vi "AlazarBusy.vi"(0 "Handle":u64, 1 "error in (no error)":errorcluster) -> (2 "Handle":u64, 3 "Busy":bool, 4 "Return Code":u32, 5 "error out":errorcluster)   [LabVIEW 2018]
doc: "Determine if an acquisition to on-board memory is in progress."
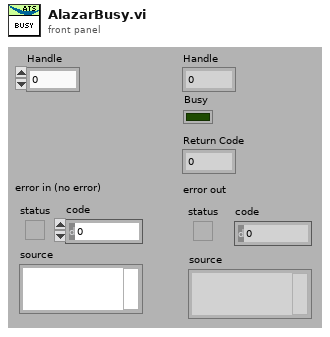
[diagram p1: front panel]
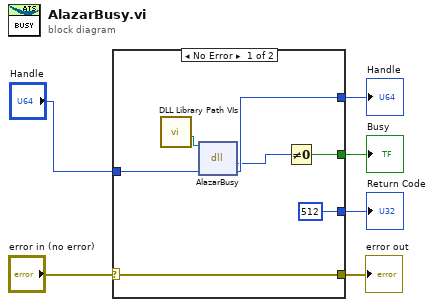
[diagram p0: block diagram]
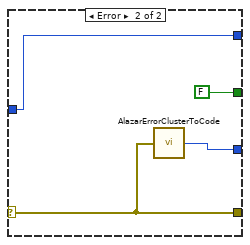
[diagram p2: hidden frame]
diagram:
  n1 = case shown="No Error" "error in (no error)" {
    selector: "error in (no error)" -> [w10 w17]
    tunnel: [w10 w17] -> w5
    tunnel: [u32 512 w16] -> w4
    tunnel: "Handle" -> [w13 w15]
    tunnel: [w12 w15] -> w2
    tunnel: [w8 FALSE] -> w1
    frame No Error {
      n2 = call "DLL Library Path VIs.vi"() -> ("Alazar"=w7:path)  [unwired: 9 in, 2 out]
      n3 = dll-call lib="C:/Project/SerialSectOCT - FFT GPU/SerialSectOCT/Labview Software/DLL/ATSApi.dll" fn="AlazarBusy"(path in=w7, "handle"=w13) -> ("return type"=w9:u32, "handle"=w12:u64)  [unwired: 2 in, 2 out]
      n4 = Not Equal To 0?(x=w9) -> (x != 0?=w8:bool)
    }
    frame Error {
      n5 = call "AlazarErrorClusterToCode.vi"("error in (no error)"=w17) -> ("Error Code"=w16:u32)
    }
  }
  "Handle" <- w2
  "error out" <- w5
  "Return Code" <- w4
  "Busy" <- w1
